vi "acquisition multipoint CEL1.vi"(7 "nb mur HP1":i32, 8 "entrée d'erreur":errorcluster, 9 "Cluster VISA":T3, 10 "Cluster voies acquisition":T2, 11 "cluster donnée":T1) -> (0 "sortie d'erreur":errorcluster, 3 "chaine data":string)   [LabVIEW 2017]
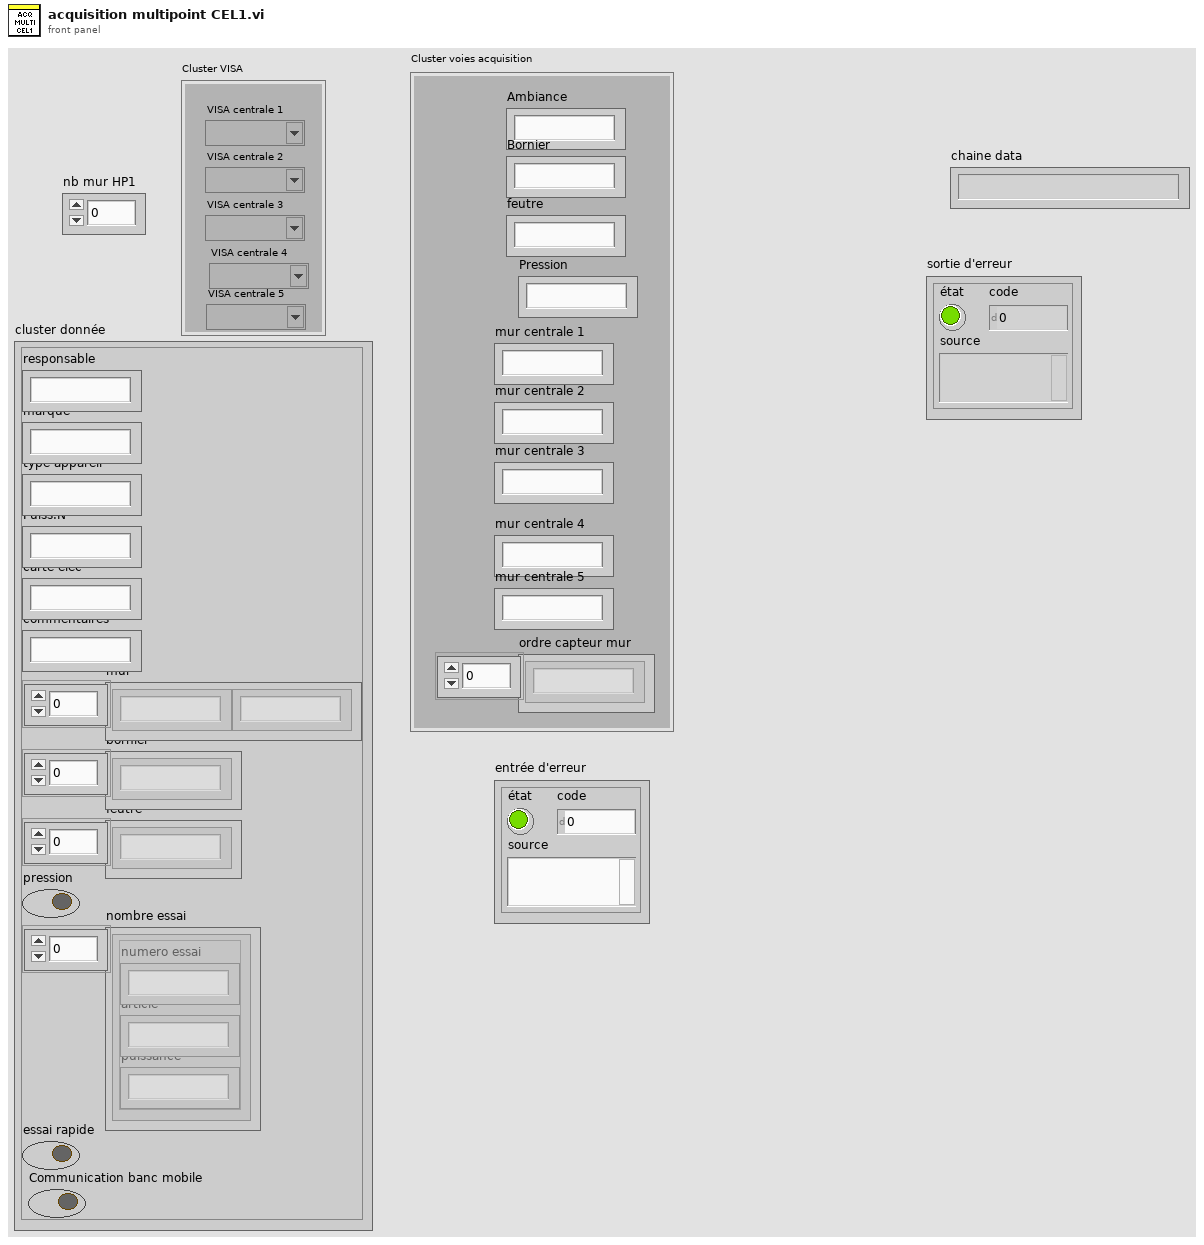
[diagram p1: front panel]
types:
  T1 = cluster{"responsable":string, "marque":string, "type appareil":string, "Puiss.N":string, "carte élec":string, "commentaires":string, "mur":string[], "bornier":string[], "feutre":string[], "pression":bool, "nombre essai":cluster{"numero essai":string, "article":string, "puissance":string}[], "essai rapide":bool, "Communication banc mobile":bool}
  T2 = cluster{"Ambiance":string, "Bornier":string, "feutre":string, "Pression":string, "mur centrale 1":string, "mur centrale 2":string, "mur centrale 3":string, "mur centrale 4":string, "mur centrale 5":string, "ordre capteur mur":string[]}
  T3 = cluster{"VISA centrale 1":refnum<visa-resource-name>, "VISA centrale 2":refnum<visa-resource-name>, "VISA centrale 3":refnum<visa-resource-name>, "VISA centrale 4":refnum<visa-resource-name>, "VISA centrale 5":refnum<visa-resource-name>}
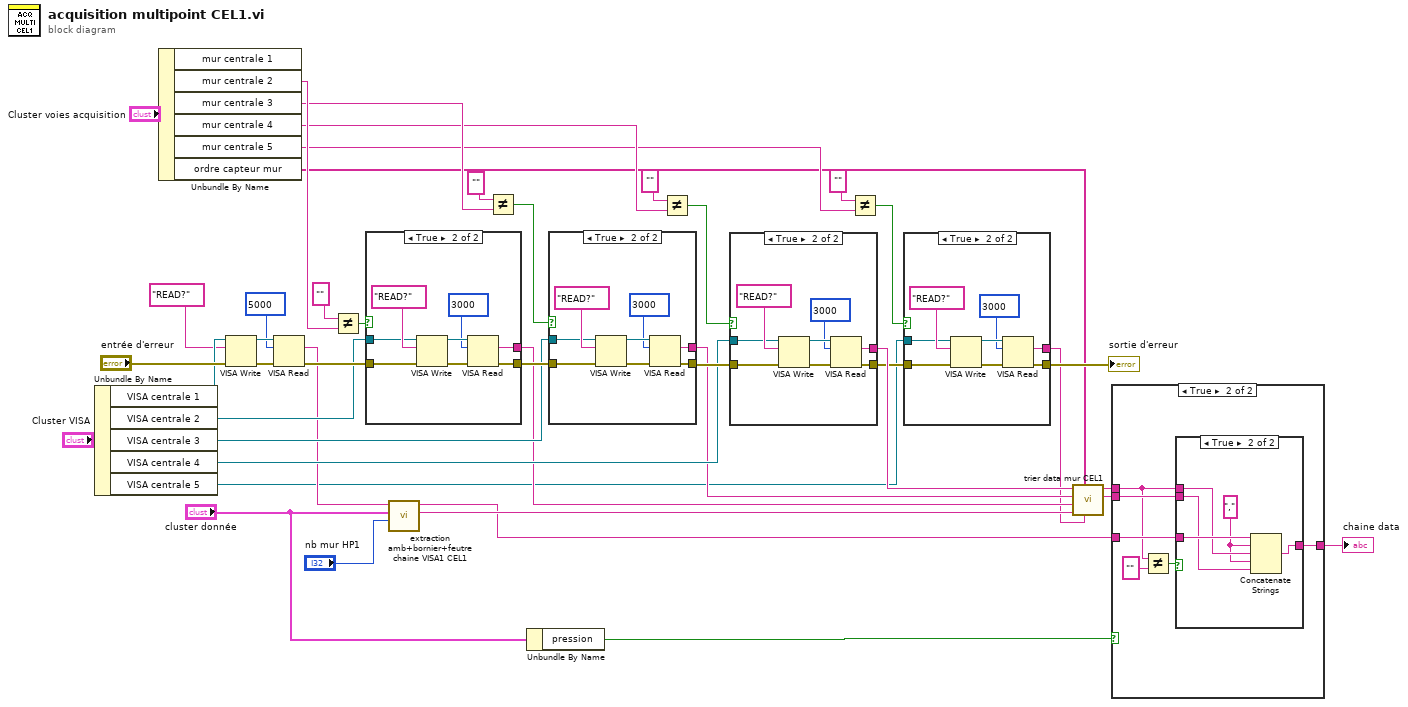
[diagram p0: block diagram]
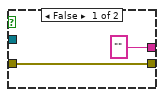
[diagram p2: hidden frame]
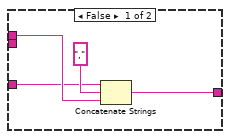
[diagram p3: hidden frame]
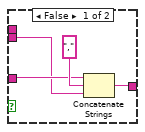
[diagram p4: hidden frame]
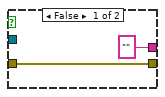
[diagram p5: hidden frame]
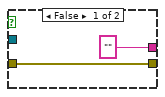
[diagram p6: hidden frame]
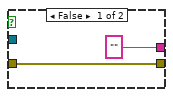
[diagram p7: hidden frame]
diagram:
  n1 = Unbundle By Name("Cluster VISA") -> ("VISA centrale 1"=w40:refnum<visa-resource-name>, "VISA centrale 2"=w23:refnum<visa-resource-name>, "VISA centrale 3"=w22:refnum<visa-resource-name>, "VISA centrale 4"=w21:refnum<visa-resource-name>, "VISA centrale 5"=w5:refnum<visa-resource-name>)
  n2 = Unbundle By Name("Cluster voies acquisition") -> ("mur centrale 2"=w33:string, "mur centrale 3"=w28:string, "mur centrale 4"=w24:string, "mur centrale 5"=w3:string, "ordre capteur mur"=w2:string[])  [unwired: 1 out]
  n3 = VISA Write(VISA resource name=w40, write buffer="READ?" ("buffer d'écriture"), error in (no error)="entrée d'erreur") -> (VISA resource name out=w38:refnum<visa-resource-name>, error out=w41:errorcluster)  [unwired: 1 out]
  n4 = VISA Read(VISA resource name=w38, byte count=u32 5000 ("nombre d'octets"), error in (no error)=w41) -> (read buffer=w20:string, error out=w36:errorcluster)  [unwired: 2 out]
  n5 = Not Equal?(x="", y=w33) -> (x != y?=w35:bool)
  n6 = case shown="True" w35 {
    tunnel: w36 -> [w45 w49]
    tunnel: ["" ("read buffer") w48] -> w17
    tunnel: [w45 w47] -> w31
    tunnel: w23 -> [_ w46]
    frame False {
    }
    frame True {
      n7 = VISA Write(VISA resource name=w46, write buffer="READ?" ("buffer d'écriture"), error in (no error)=w49) -> (VISA resource name out=w51:refnum<visa-resource-name>, error out=w53:errorcluster)  [unwired: 1 out]
      n8 = VISA Read(VISA resource name=w51, byte count=u32 3000 ("nombre d'octets"), error in (no error)=w53) -> (read buffer=w48:string, error out=w47:errorcluster)  [unwired: 2 out]
    }
  }
  n9 = call "extraction amb+bornier+feutre chaine VISA1 CEL1.vi"("nb mur HP1"="nb mur HP1", "cluster donnée"="cluster donnée", "buffer lecture VISA 1"=w20) -> ("chaine mur+pression"=w16:string, "chaine amb+bornier+feutre"=w15:string)  [unwired: 7 in]
  n10 = Not Equal?(x="", y=w28) -> (x != y?=w29:bool)
  n11 = Unbundle By Name("cluster donnée") -> ("pression"=w11:bool)
  n12 = case shown="True" w29 {
    tunnel: w31 -> [w55 w59]
    tunnel: ["" ("read buffer") w58] -> w18
    tunnel: [w55 w57] -> w26
    tunnel: w22 -> [_ w56]
    frame False {
    }
    frame True {
      n13 = VISA Write(VISA resource name=w56, write buffer="READ?" ("buffer d'écriture"), error in (no error)=w59) -> (VISA resource name out=w61:refnum<visa-resource-name>, error out=w63:errorcluster)  [unwired: 1 out]
      n14 = VISA Read(VISA resource name=w61, byte count=u32 3000 ("nombre d'octets"), error in (no error)=w63) -> (read buffer=w58:string, error out=w57:errorcluster)  [unwired: 2 out]
    }
  }
  n15 = Not Equal?(x="", y=w24) -> (x != y?=w25:bool)
  n16 = case shown="True" w25 {
    tunnel: w26 -> [w65 w69]
    tunnel: ["" ("read buffer") w68] -> w19
    tunnel: [w65 w67] -> w9
    tunnel: w21 -> [_ w66]
    frame False {
    }
    frame True {
      n17 = VISA Write(VISA resource name=w66, write buffer="READ?" ("buffer d'écriture"), error in (no error)=w69) -> (VISA resource name out=w71:refnum<visa-resource-name>, error out=w73:errorcluster)  [unwired: 1 out]
      n18 = VISA Read(VISA resource name=w71, byte count=u32 3000 ("nombre d'octets"), error in (no error)=w73) -> (read buffer=w68:string, error out=w67:errorcluster)  [unwired: 2 out]
    }
  }
  n19 = Not Equal?(x="", y=w3) -> (x != y?=w6:bool)
  n20 = case shown="True" w6 {
    tunnel: w9 -> [w75 w79]
    tunnel: ["" ("read buffer") w78] -> w4
    tunnel: [w75 w77] -> w8
    tunnel: w5 -> [_ w76]
    frame False {
    }
    frame True {
      n21 = VISA Write(VISA resource name=w76, write buffer="READ?" ("buffer d'écriture"), error in (no error)=w79) -> (VISA resource name out=w81:refnum<visa-resource-name>, error out=w83:errorcluster)  [unwired: 1 out]
      n22 = VISA Read(VISA resource name=w81, byte count=u32 3000 ("nombre d'octets"), error in (no error)=w83) -> (read buffer=w78:string, error out=w77:errorcluster)  [unwired: 2 out]
    }
  }
  "sortie d'erreur" <- w8
  n23 = call "trier data mur CEL1.vi"("data VISA 5"=w4, "ordre capteur mur"=w2, "data VISA 1"=w16, "data VISA 2"=w17, "data VISA 3"=w18, "data VISA 4"=w19) -> ("data pression"=w13:string, "data mur"=w14:string)  [unwired: 4 in]
  n24 = case shown="True" w11 {
    tunnel: w15 -> [w85 w93]
    tunnel: w14 -> [w86 w89]
    tunnel: w13 -> [_ w92]
    tunnel: [w84 w91] -> w10
    frame False {
      n25 = Concatenate Strings(w85, ",", w86) -> (w84:string)
    }
    frame True {
      n26 = Not Equal?(x=w89, y="") -> (x != y?=w90:bool)
      n27 = case shown="True" w90 {
        tunnel: w93 -> [w95 w102]
        tunnel: w89 -> [_ w101]
        tunnel: w92 -> [w94 w100]
        tunnel: [w96 w98] -> w91
        frame False {
          n28 = Concatenate Strings(w95, ",", w94) -> (w96:string)
        }
        frame True {
          w99 = ","
          n29 = Concatenate Strings(w102, w99, w101, w99, w100) -> (w98:string)
        }
      }
    }
  }
  "chaine data" <- w10
